vi "LC DB Query.vi"(7 "Read?":bool, 8 "error in (no error)":errorcluster caption="Error In", 10 "SQL query":string, 11 "DB Ref In":T1) -> (0 "error out":errorcluster caption="Error Out", 2 "Data":string[][](array[string]), 3 "DB Ref Out":T1)   [LabVIEW 2020]
uses:
  <vilib>/addons/database/Connection.llb/Conn ObjectReference.ctl
  <vilib>/addons/database/Connection.llb/Conn Execute.vi
  <vilib>/addons/database/Recordset.llb/Rec Fetch Recordset Data (R).vi
  <vilib>/addons/database/Recordset.llb/Rec Destroy - Connection.vi
  <vilib>/addons/database/_DB Variant To Data/Database Variant To Data.xnode
  <vilib>/addons/database/NI_Database_API.lvlib
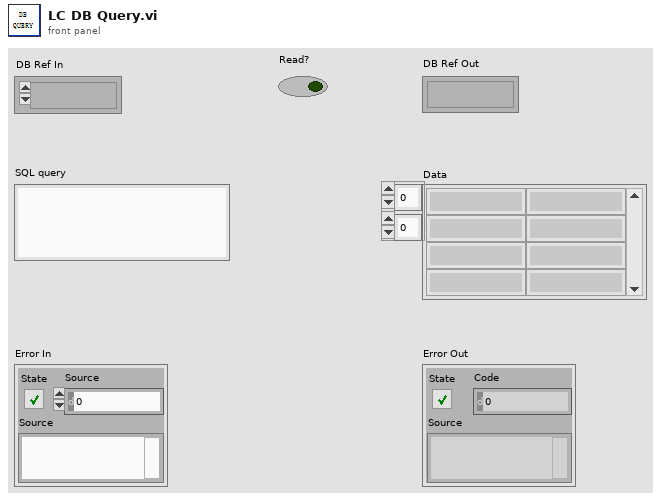
[diagram p1: front panel]
types:
  T1 = typedef "NI_Database_API.lvlib/Conn ObjectReference.ctl" = refnum<k1>
  T2 = typedef "NI_Database_API.lvlib/Rec ObjectReference.ctl" = refnum<k1>
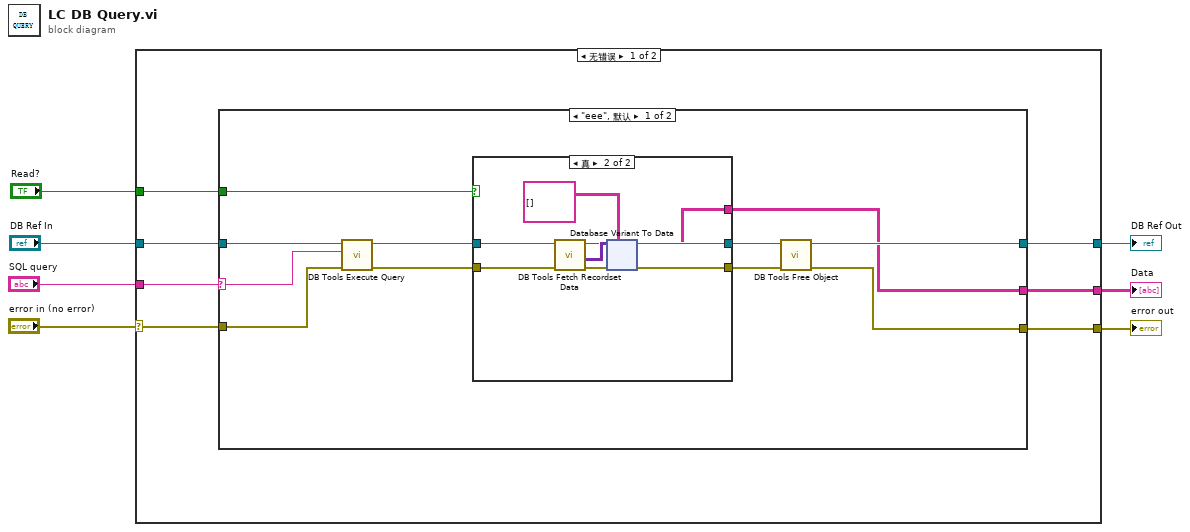
[diagram p0: block diagram]
diagram:
  n1 = case shown="无错误" "error in (no error)" {
    selector: "error in (no error)" -> [w12 w82]
    tunnel: "DB Ref In" -> [w14 w83]
    tunnel: [w13 w83] -> w2
    tunnel: [w11 w82] -> w4
    tunnel: "SQL query" -> [w10 _]
    tunnel: [w9 _] -> w6
    tunnel: "Read?" -> [w8 _]
    frame No Error {
      n2 = case shown="\"eee\", 默认" w10 {
        selector: w10 -> [w17 _]
        tunnel: w14 -> [w21 w81]
        tunnel: [w20 w81] -> w13
        tunnel: w12 -> [w19 w80]
        tunnel: [w18 w80] -> w11
        tunnel: [w16 _] -> w9
        tunnel: w8 -> [w15 _]
        frame "eee", Default {
          n3 = call-poly <vilib>:"DB Tools Execute Query.vi"("error in (no error)"=w19, "SQL query"=w17, "connection reference"=w21) -> ("error out"=w24:errorcluster, "recordset reference"=w25:T2)  [unwired: 5 in]
          n4 = case shown="真" w15 {
            tunnel: w25 -> [w27 w35]
            tunnel: w24 -> [w26 w34]
            tunnel: [w26 w32] -> w23
            tunnel: [w27 w30] -> w22
            tunnel: [_ w28] -> w16
            frame False {
            }
            frame True {
              n5 = call-poly <vilib>:"DB Tools Fetch Recordset Data.vi"("error in (no error)"=w34, "recordset reference"=w35) -> ("error out"=w33:errorcluster, "recordset data"=w31:variant[][], "recordset reference out"=w30:T2)  [unwired: 3 in]
              n6 = xnode "Database Variant To Data"("database variant"=w31, "error in (no error)"=w33, "type"=string[][] []) -> ("data"=w28:string[][], "error out"=w32:errorcluster)
            }
          }
          n7 = call-poly <vilib>:"DB Tools Free Object.vi"("error in (no error)"=w23, "recordset reference"=w22) -> ("error out"=w18:errorcluster, "connection reference"=w20:T1)  [unwired: 8 in]
        }
        frame "" {
        }
      }
    }
    frame Error {
    }
  }
  "DB Ref Out" <- w2
  "error out" <- w4
  "Data" <- w6
